vi "Start Haptic Loop.vi"(8 "error in (no error)":errorcluster, 10 "Mode Selection":u16(ring) items=["Custom Mode", "Read Mode", "STM Write Mode", "AFM Write Mode"]) -> (0 "error out":errorcluster)   [LabVIEW 2019, in "Haptic Prog Interface.lvlib"]
doc: "Begins the haptic loop, must be ran before any other VI from the library is ran."
uses:
  Haptic Prog Interface.lvlib
  dll_path.vi
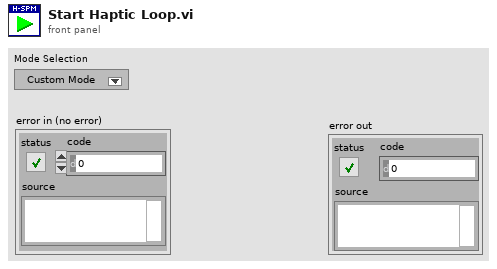
[diagram p1: front panel]
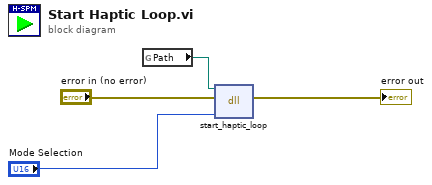
[diagram p0: block diagram]
diagram:
  n1 = global read "dll_path.vi" "Path"() -> (w4:path)
  n2 = dll-call lib="C:/Users/freem/Documents/GitHub/HapticSPM/Haptic-Programming-Interface/x64/Release/Haptic Programming Interface.dll" fn="start_haptic_loop"(path in=w4, error in="error in (no error)", "input"="Mode Selection") -> (error out=→"error out":errorcluster)  [unwired: 3 in, 1 out]
